vi "ABD_Compute.vi"(8 "error in":errorcluster, 11 "Model Data":T2 {"Matricies"."K" format="%#_6e"; "Matricies"."Dout" format="%#_6e"; "Matricies"."Bout" format="%#_6e"; "Matricies"."Aout" format="%#_6e"; "Matricies"."Dint" format="%#_6e"; "Matricies"."Bint" format="%#_6e"; "Matricies"."Aint" format="%#_6e"; "Constants"."Z" format="%^#_6e"}) -> (0 "error out":errorcluster, 3 "Model Data out":T2 {"Matricies"."K" format="%#_6e"; "Matricies"."Dout" format="%#_6e"; "Matricies"."Bout" format="%#_6e"; "Matricies"."Aout" format="%#_6e"; "Matricies"."Dint" format="%#_6e"; "Matricies"."Bint" format="%#_6e"; "Matricies"."Aint" format="%#_6e"; "Constants"."Z" format="%^#_6e"})   [LabVIEW 2012]
uses:
  Model Data.ctl
  PZT type.ctl
  Piezo_Discs.ctl
  LEM_Params.ctl
  Layer Properties.ctl
  Matricies.ctl
panel:
  out "Mr":dbl
  out "Nr":dbl
  out "Matricies":T1 {"K" format="%#_6e"; "Dout" format="%#_6e"; "Bout" format="%#_6e"; "Aout" format="%#_6e"; "Dint" format="%#_6e"; "Bint" format="%#_6e"; "Aint" format="%#_6e"}
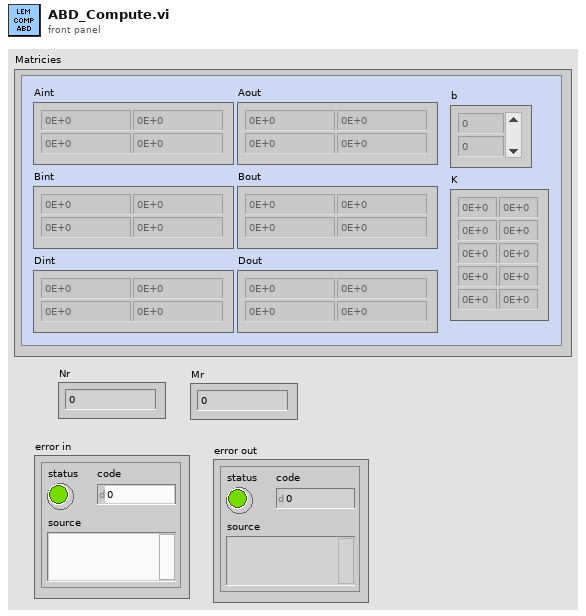
[diagram p1: front panel]
types:
  T1 = typedef "Matricies.ctl" = cluster{"Aint":dbl[][], "Bint":dbl[][], "Dint":dbl[][], "Aout":dbl[][], "Bout":dbl[][], "Dout":dbl[][], "b":dbl[], "K":dbl[][]}
  T2 = typedef "Model Data.ctl" = cluster{"Disc Properties":cluster{"Type":T3, "Disc Model":T4}, "Constants":cluster{"Radius":dbl[], "U(r)":dbl[], "W(r)":dbl[], "Vac":dbl, "P":dbl, "RiRo":dbl, "Area Density (r)":dbl[], "Ro":dbl, "Ri":dbl, "Z":dbl[], "Nr":dbl, "Mr":dbl, "c":dbl[], "AoC":dbl, "BoC":dbl, "AiC":dbl, "BiC":dbl, "f1":dbl, "f2":dbl}, "LEM Parameters":T5, "Layer Properties":T6[], "Matricies":T1}
  T3 = typedef "PZT type.ctl" = enum16{"Bimorph", "Unimorph"}
  T4 = typedef "Piezo_Discs.ctl" = enum16{"FTBD-21T-4.0A1", "PZT-5A (Gallas 1)", "PZT-5A (Gallas 2)", "AB4113B", "Create new disc...", "Load disc from file..."}
  T5 = typedef "LEM_Params.ctl" = cluster{"Displacement Ratio":dbl, "Cd":dbl, "Md":dbl, "xdc":dbl, "fd":dbl, "Sensitivity":dbl, "dA":dbl, "Rd":dbl, "Zeta":dbl, "Phi":dbl}
  T6 = typedef "Layer Properties.ctl" = cluster{"E":dbl, "R":dbl, "rho":dbl, "rhoA":dbl, "v":dbl, "A":dbl, "t":dbl, "d31":dbl, "size":enum16{"Outer", "Inner"}}
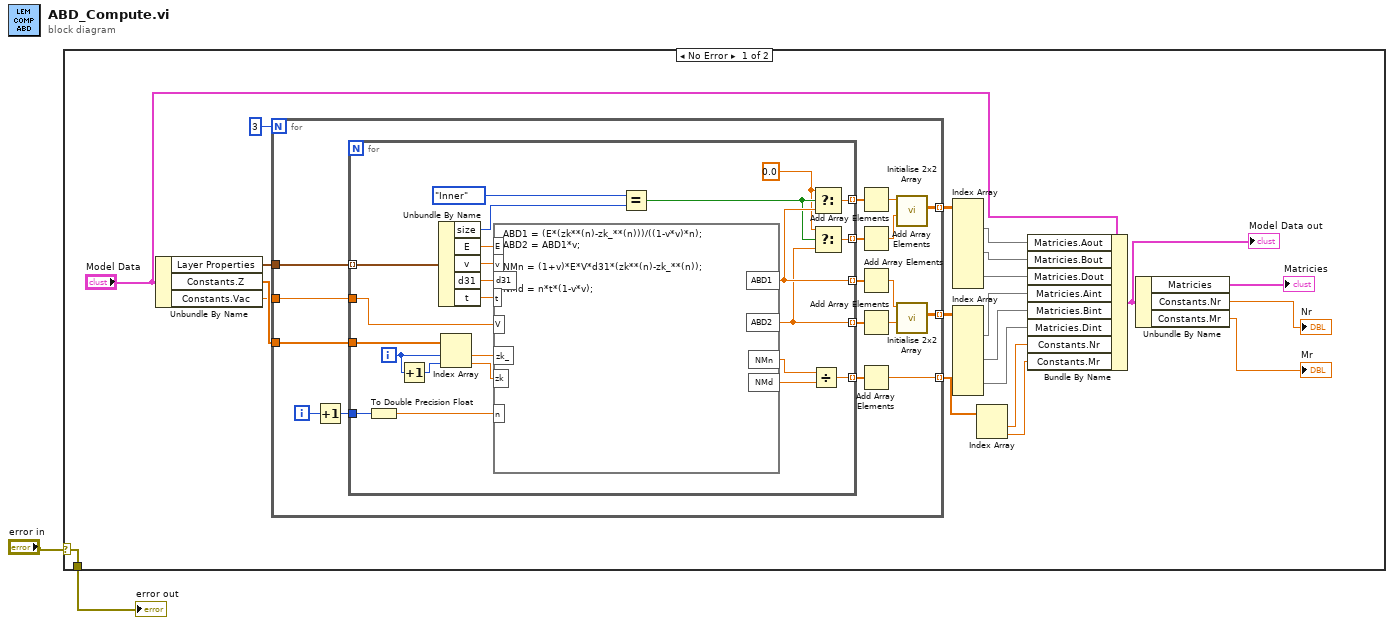
[diagram p0: block diagram]
diagram:
  n1 = case shown="No Error" "error in" {
    selector: "error in" -> [w3 w65]
    tunnel: [w3 w65] -> w1
    frame No Error {
      n2 = Unbundle By Name("Model Data") -> ("Layer Properties"=w20:T6[], "Constants.Z"=w19:dbl[], "Constants.Vac"=w9:dbl)
      n3 = for {
        N: 3 -> [_]
        tunnel: w20 -> [w40]
        tunnel: w19 -> [w39]
        tunnel: [w30] -> w18 mode=indexing
        tunnel: [w29] -> w14 mode=indexing
        tunnel: w9 -> [w26]
        tunnel: [w24] -> w4 mode=indexing
        i -> [w28]
        n4 = Increment(x=w28) -> (x+1=w27:i32)
        n5 = for {
          tunnel: w40 -> [w64] mode=indexing
          tunnel: w39 -> [w63]
          tunnel: w27 -> [w47]
          tunnel: [w53] -> w36 mode=indexing
          tunnel: [w50] -> w35 mode=indexing
          tunnel: [w52] -> w38 mode=indexing
          tunnel: [w49] -> w37 mode=indexing
          tunnel: w26 -> [w45]
          tunnel: [w41] -> w25 mode=indexing
          i -> [w62]
          w48 = 0.0 ("t")
          n6 = To Double Precision Float(number=w47) -> (double precision float=w60:dbl)
          n7 = Increment(x=w62) -> (x+1=w61:i32)
          n8 = Unbundle By Name(w64) -> ("size"=w55:enum16{"Outer", "Inner"}, "E"=w56:dbl, "v"=w57:dbl, "d31"=w46:dbl, "t"=w44:dbl)
          n9 = Index Array(array=w63, index #1=w62, index #2=w61) -> (element #1=w58:dbl, element #2=w59:dbl)
          n10 = formula code="ABD1 = (E*(zk**(n)-zk_**(n)))/((1-v*v)*n);\nABD2 = ABD1*v;\n\nNMn = (1+v)*E*V*d31*(zk**(n)-zk_**(n));\n\nNMd = n*t*(1-v*v);"("E"=w56, "v"=w57, "zk_"=w58, "zk"=w59, "n"=w60, "d31"=w46, "V"=w45, "t"=w44) -> ("ABD1"=w53:dbl, "ABD2"=w50:dbl, "NMn"=w42:dbl, "NMd"=w43:dbl)
          n11 = Equal?(x=enum16{"Outer", "Inner"}."Inner", y=w55) -> (x = y?=w51:bool)
          n12 = Divide(x=w42, y=w43) -> (x/y=w41:dbl)
          n13 = Select(t=w48, s=w51, f=w53) -> (s? t:f=w52:dbl)
          n14 = Select(t=w48, s=w51, f=w50) -> (s? t:f=w49:dbl)
        }
        n15 = Add Array Elements(numeric array=w38) -> (sum=w34:dbl)
        n16 = Add Array Elements(numeric array=w37) -> (sum=w33:dbl)
        n17 = Add Array Elements(numeric array=w36) -> (sum=w32:dbl)
        n18 = Add Array Elements(numeric array=w35) -> (sum=w31:dbl)
        n19 = Add Array Elements(numeric array=w25) -> (sum=w24:dbl)
        n20 = call "Initialise 2x2 Array.vi"("element"=w33, "new diagonal/fill element"=w34) -> ("Output Array"=w30:dbl[][])  [unwired: 9 in]
        n21 = call "Initialise 2x2 Array.vi"("element"=w31, "new diagonal/fill element"=w32) -> ("Output Array"=w29:dbl[][])  [unwired: 9 in]
      }
      n22 = Index Array(array=w18) -> (element #1=w17:dbl[][], element #2=w16:dbl[][], element #3=w15:dbl[][])  [unwired: 9 in]
      n23 = Index Array(array=w14) -> (element #1=w13:dbl[][], element #2=w12:dbl[][], element #3=w11:dbl[][])  [unwired: 9 in]
      n24 = Index Array(array=w4) -> (element #1=w8:dbl, element #2=w7:dbl)  [unwired: 2 in]
      n25 = Bundle By Name(cluster="Model Data", "Matricies.Aout"=w17, "Matricies.Bout"=w16, "Matricies.Dout"=w15, "Matricies.Aint"=w13, "Matricies.Bint"=w12, "Matricies.Dint"=w11, "Constants.Nr"=w8, "Constants.Mr"=w7) -> (w22:T2)
      "Model Data out" <- w22
      n26 = Unbundle By Name(w22) -> ("Matricies"=→"Matricies":T1, "Constants.Nr"=→"Nr":dbl, "Constants.Mr"=→"Mr":dbl)
    }
    frame Error {
    }
  }
  "error out" <- w1
